vi "Get SerialNumber.vi"(8 "error in (no error)":errorcluster, 11 "TLCamera reference in":refnum<k24>) -> (0 "error out":errorcluster, 2 "SerialNumber":string, 3 "TLCamera reference out":refnum<k24>)   [LabVIEW 2015]
uses:
  C:/code/Host/Installer/Scientific Camera Interfaces/LabVIEW/64_bit/Library_X64/Thorlabs.TSI.TLCameraInterfaces.dll
  code/Host/Installer/Scientific Camera Interfaces/LabVIEW/64_bit/Library_X64/Thorlabs.TSI.TLCameraInterfaces.dll
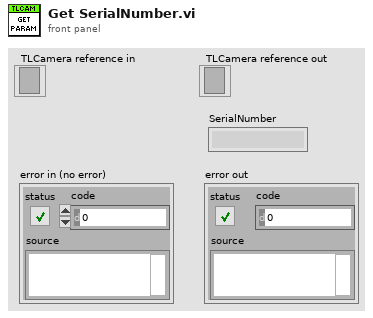
[diagram p1: front panel]
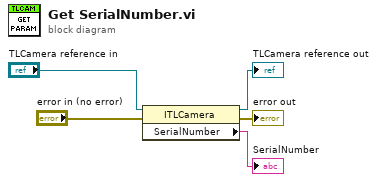
[diagram p0: block diagram]
diagram:
  n1 = property class="ITLCamera"(reference="TLCamera reference in", error in="error in (no error)") -> (reference out=→"TLCamera reference out":refnum<k24>, error out=→"error out":errorcluster, "SerialNumber"=→"SerialNumber":string)
